vi "FTW-Panel-EnableControl.vi"(7 "Enable?":bool) -> (8 "Control Enabled State":T1(ring))   [LabVIEW 2013]
panel:
  # "Inputs"
  # "Outputs"
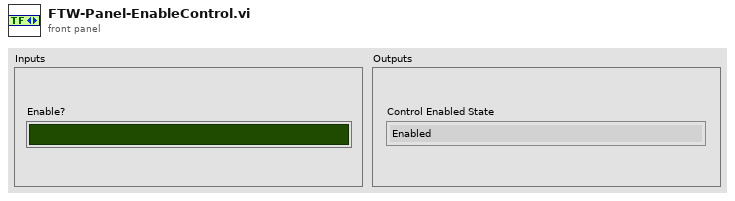
[diagram p1: front panel]
types:
  T1 = enum8{"Enabled", "Disabled", "Disabled and Grayed Out"}
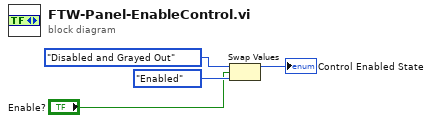
[diagram p0: block diagram]
diagram:
  n1 = Swap Values(12:T1."Disabled and Grayed Out" ("Disabled"), 13:"Enable?", 14:T1."Enabled" ("Disabled")) -> (1:→"Control Enabled State":T1)  [unwired: 1 out]
